vi "CellClicked Event Callback.vi"(4 "DataGridView in":refnum<class "DataGridView.lvclass">, 5 "Event Data":cluster{"sender":refnum<k24>, "e":refnum<k24>}, 6 "Control Ref":refnum<k24>, 7 "Event Common Data":T1) -> ()   [LabVIEW 2020, in "DataGrid.lvlib" / "DataGridView.lvclass"]
doc: "When a cell is clicked, the user event returns the row and index clicked."
uses:
  DataGridView/DataGridView.lvclass
  System.Windows.Forms
  CellClick/CellClick.lvclass
  C:/GEECS/Developers Version/source/Shared/LabVIEWdotNetDataGrid-master/source/Events/Abstract EVENT/Abstract EVENT.lvclass
  CellClick/CellClick.lvclass/CellClick.ctl
  CellClick/Write row.vi
  CellClick/Write column.vi
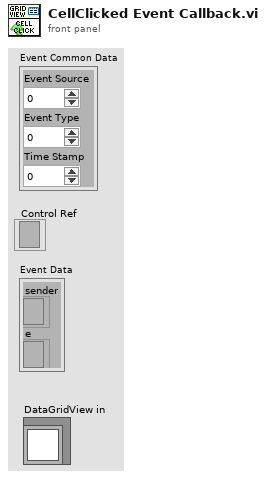
[diagram p1: front panel]
types:
  T1 = cluster{"Event Source":i32, "Event Type":u32, "Time Stamp":u32}
  T2 = cluster{"CellClicked":refnum<user-event>, "CellValue Changed":refnum<user-event>, "KeyDown":refnum<user-event>, "DataError":refnum<user-event>, "UserAddedRow":refnum<user-event>, "UserDeletedRow":refnum<user-event>, "CellDirtyStateChanged":refnum<user-event>}
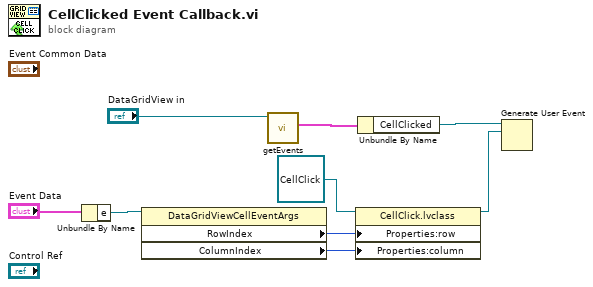
[diagram p0: block diagram]
diagram:
  n1 = Unbundle By Name("Event Data") -> ("e"=w3:refnum<k24>)
  n2 = property class="DataGridViewCellEventArgs"(reference=w3) -> ("RowIndex"=w2:i32, "ColumnIndex"=w1:i32)  [unwired: 1 in, 2 out]
  n3 = call "getEvents.vi"("DataGridView in"="DataGridView in") -> ("userEvents"=w5:T2)  [unwired: 8 in, 2 out]
  n4 = property class="CellClick.lvclass"(reference=refnum<class "CellClick.lvclass"> refnum ("DataGrid.lvlib:CellClick.lvclass"), "Properties:row"=w2, "Properties:column"=w1) -> (reference out=w7:refnum<class "CellClick.lvclass">)  [unwired: 1 in, 1 out]
  n5 = Unbundle By Name(w5) -> ("CellClicked"=w4:refnum<user-event>)
  n6 = Generate User Event(user event=w4, event data cluster=w7) -> ()  [unwired: 2 in, 2 out]
